vi "CreateEventTypeEnum.vi"() -> ()   [LabVIEW 2024]
uses:
  <vilib>/Utility/error.llb/Trim Whitespace One-Sided.vi
  SDL3/Events/EventType--enum.ctl
  <vilib>/regexp/Match Regular Expression.xnode
  SDL3/Events/Events.lvlib
panel:
  out "delimited string":string
  in  "#Define list":string="SDL_EVENT_QUIT           = 0x100, /**< User-requested quit */\n\n\n    SDL_EVENT_LOCALE_CHANGED,  /**< The user's locale preferences have changed. */\n\n    SDL_EVENT_SYSTEM_THEME_CHANGED, /**< The system theme changed */\n\n    SDL_EVENT_DISPLAY_ORIENTATION = 0x151,   /**< Display orientation has changed to data1 */\n    SDL_EVENT_DISPLAY_ADDED,                 /**< Display has been added to the system */\n    SDL_EVENT_DISPLAY_REMOVED,               /**< Display has been removed from the system */\n    SDL_EVENT_DISPLAY_MOVED,                 /**< Display has changed position */\n    SDL_EVENT_DISPLAY_DESKTOP_MODE_CHANGED,  /**< Display has changed desktop mode */\n    SDL_EVENT_DISPLAY_CURRENT_MODE_CHANGED,  /**< Display has changed current mode */\n    SDL_EVENT_DISPLAY_CONTENT_SCALE_CHANGED, /**< Display has changed content scale */\n\n\n\n    SDL_EVENT_WINDOW_SHOWN = 0x202,     /**< Window has been shown */\n    SDL_EVENT_WINDOW_HIDDEN,            /**< Window has been hidden */\n    SDL_EVENT_WINDOW_EXPOSED,           /**< Window has been exposed and should be redrawn, and can be redrawn directly from event watchers for this event */\n    SDL_EVENT_WINDOW_MOVED,             /**< Window has been moved to data1, data2 */\n    SDL_EVENT_WINDOW_RESIZED,           /**< Window has been resized to data1xdata2 */\n    SDL_EVENT_WINDOW_PIXEL_SIZE_CHANGED,/**< The pixel size of the window has changed to data1xdata2 */\n    SDL_EVENT_WINDOW_METAL_VIEW_RESIZED,/**< The pixel size of a Metal view associated with the window has changed */\n    SDL_EVENT_WINDOW_MINIMIZED,         /**< Window has been minimized */\n    SDL_EVENT_WINDOW_MAXIMIZED,         /**< Window has been maximized */\n    SDL_EVENT_WINDOW_RESTORED,          /**< Window has been restored to normal size and position */\n    SDL_EVENT_WINDOW_MOUSE_ENTER,       /**< Window has gained mouse focus */\n    SDL_EVENT_WINDOW_MOUSE_LEAVE,       /**< Window has lost mouse focus */\n    SDL_EVENT_WINDOW_FOCUS_GAINED,      /**< Window has gained keyboard focus */\n    SDL_EVENT_WINDOW_FOCUS_LOST,        /**< Window has lost keyboard focus */\n    SDL_EVENT_WINDOW_CLOSE_REQUESTED,   /**< The window manager requests that the window be closed */\n    SDL_EVENT_WINDOW_HIT_TEST,          /**< Window had a hit test that wasn't SDL_HITTEST_NORMAL */\n    SDL_EVENT_WINDOW_ICCPROF_CHANGED,   /**< The ICC profile of the window's display has changed */\n    SDL_EVENT_WINDOW_DISPLAY_CHANGED,   /**< Window has been moved to display data1 */\n    SDL_EVENT_WINDOW_DISPLAY_SCALE_CHANGED, /**< Window display scale has been changed */\n    SDL_EVENT_WINDOW_SAFE_AREA_CHANGED, /**< The window safe area has been changed */\n    SDL_EVENT_WINDOW_OCCLUDED,          /**< The window has been occluded */\n    SDL_EVENT_WINDOW_ENTER_FULLSCREEN,  /**< The window has entered fullscreen mode */\n    SDL_EVENT_WINDOW_LEAVE_FULLSCREEN,  /**< The window has left fullscreen mode */\n    SDL_EVENT_WINDOW_DESTROYED,         /**< The window with the associated ID is being or has been destroyed. If this message is being handled in an event watcher, the window handle is still valid and can still be used to retrieve any properties associated with the window. Otherwise, the handle has already been destroyed and all resources associated with it are invalid */\n    SDL_EVENT_WINDOW_HDR_STATE_CHANGED, /**< Window HDR properties have changed */\n\n\n\n    SDL_EVENT_KEY_DOWN        = 0x300, /**< Key pressed */\n    SDL_EVENT_KEY_UP,                  /**< Key released */\n    SDL_EVENT_TEXT_EDITING,            /**< Keyboard text editing (composition) */\n    SDL_EVENT_TEXT_INPUT,              /**< Keyboard text input */\n    SDL_EVENT_KEYMAP_CHANGED,          /**< Keymap changed due to a system event such as an input language or keyboard layout change. */\n    SDL_EVENT_KEYBOARD_ADDED,          /**< A new keyboard has been inserted into the system */\n    SDL_EVENT_KEYBOARD_REMOVED,        /**< A keyboard has been removed */\n    SDL_EVENT_TEXT_EDITING_CANDIDATES, /**< Keyboard text editing candidates */\n\n\n    SDL_EVENT_MOUSE_MOTION    = 0x400, /**< Mouse moved */\n    SDL_EVENT_MOUSE_BUTTON_DOWN,       /**< Mouse button pressed */\n    SDL_EVENT_MOUSE_BUTTON_UP,         /**< Mouse button released */\n    SDL_EVENT_MOUSE_WHEEL,             /**< Mouse wheel motion */\n    SDL_EVENT_MOUSE_ADDED,             /**< A new mouse has been inserted into the system */\n    SDL_EVENT_MOUSE_REMOVED,           /**< A mouse has been removed */\n\n\n    SDL_EVENT_JOYSTICK_AXIS_MOTION  = 0x600, /**< Joystick axis motion */\n    SDL_EVENT_JOYSTICK_BALL_MOTION,          /**< Joystick trackball motion */\n    SDL_EVENT_JOYSTICK_HAT_MOTION,           /**< Joystick hat position change */\n    SDL_EVENT_JOYSTICK_BUTTON_DOWN,          /**< Joystick button pressed */\n    SDL_EVENT_JOYSTICK_BUTTON_UP,            /**< Joystick button released */\n    SDL_EVENT_JOYSTICK_ADDED,                /**< A new joystick has been inserted into the system */\n    SDL_EVENT_JOYSTICK_REMOVED,              /**< An opened joystick has been removed */\n    SDL_EVENT_JOYSTICK_BATTERY_UPDATED,      /**< Joystick battery level change */\n    SDL_EVENT_JOYSTICK_UPDATE_COMPLETE,      /**< Joystick update is complete */\n\n\n    SDL_EVENT_GAMEPAD_AXIS_MOTION  = 0x650, /**< Gamepad axis motion */\n    SDL_EVENT_GAMEPAD_BUTTON_DOWN,          /**< Gamepad button pressed */\n    SDL_EVENT_GAMEPAD_BUTTON_UP,            /**< Gamepad button released */\n    SDL_EVENT_GAMEPAD_ADDED,                /**< A new gamepad has been inserted into the system */\n    SDL_EVENT_GAMEPAD_REMOVED,              /**< A gamepad has been removed */\n    SDL_EVENT_GAMEPAD_REMAPPED,             /**< The gamepad mapping was updated */\n    SDL_EVENT_GAMEPAD_TOUCHPAD_DOWN,        /**< Gamepad touchpad was touched */\n    SDL_EVENT_GAMEPAD_TOUCHPAD_MOTION,      /**< Gamepad touchpad finger was moved */\n    SDL_EVENT_GAMEPAD_TOUCHPAD_UP,          /**< Gamepad touchpad finger was lifted */\n    SDL_EVENT_GAMEPAD_SENSOR_UPDATE,        /**< Gamepad sensor was updated */\n    SDL_EVENT_GAMEPAD_UPDATE_COMPLETE,      /**< Gamepad update is complete */\n    SDL_EVENT_GAMEPAD_STEAM_HANDLE_UPDATED,  /**< Gamepad Steam handle has changed */\n\n\n    SDL_EVENT_FINGER_DOWN      = 0x700,\n    SDL_EVENT_FINGER_UP,\n    SDL_EVENT_FINGER_MOTION,\n\n\n\n\n    SDL_EVENT_CLIPBOARD_UPDATE = 0x900, /**< The clipboard or primary selection changed */\n\n\n    SDL_EVENT_DROP_FILE        = 0x1000, /**< The system requests a file open */\n    SDL_EVENT_DROP_TEXT,                 /**< text/plain drag-and-drop event */\n    SDL_EVENT_DROP_BEGIN,                /**< A new set of drops is beginning (NULL filename) */\n    SDL_EVENT_DROP_COMPLETE,             /**< Current set of drops is now complete (NULL filename) */\n    SDL_EVENT_DROP_POSITION,             /**< Position while moving over the window */\n\n\n    SDL_EVENT_AUDIO_DEVICE_ADDED = 0x1100,  /**< A new audio device is available */\n    SDL_EVENT_AUDIO_DEVICE_REMOVED,         /**< An audio device has been removed. */\n    SDL_EVENT_AUDIO_DEVICE_FORMAT_CHANGED,  /**< An audio device's format has been changed by the system. */\n\n\n    SDL_EVENT_SENSOR_UPDATE = 0x1200,     /**< A sensor was updated */\n\n\n    SDL_EVENT_PEN_PROXIMITY_IN = 0x1300,  /**< Pressure-sensitive pen has become available */\n    SDL_EVENT_PEN_PROXIMITY_OUT,          /**< Pressure-sensitive pen has become unavailable */\n    SDL_EVENT_PEN_DOWN,                   /**< Pressure-sensitive pen touched drawing surface */\n    SDL_EVENT_PEN_UP,                     /**< Pressure-sensitive pen stopped touching drawing surface */\n    SDL_EVENT_PEN_BUTTON_DOWN,            /**< Pressure-sensitive pen button pressed */\n    SDL_EVENT_PEN_BUTTON_UP,              /**< Pressure-sensitive pen button released */\n    SDL_EVENT_PEN_MOTION,                 /**< Pressure-sensitive pen is moving on the tablet */\n    SDL_EVENT_PEN_AXIS,                   /**< Pressure-sensitive pen angle/pressure/etc changed */\n\n\n    SDL_EVENT_CAMERA_DEVICE_ADDED = 0x1400,  /**< A new camera device is available */\n    SDL_EVENT_CAMERA_DEVICE_REMOVED,         /**< A camera device has been removed. */\n    SDL_EVENT_CAMERA_DEVICE_APPROVED,        /**< A camera device has been approved for use by the user. */\n    SDL_EVENT_CAMERA_DEVICE_DENIED,          /**< A camera device has been denied for use by the user. */\n\n\n    SDL_EVENT_RENDER_TARGETS_RESET = 0x2000, /**< The render targets have been reset and their contents need to be updated */\n    SDL_EVENT_RENDER_DEVICE_RESET, /**< The device has been reset and all textures need to be recreated */\n\n\n    SDL_EVENT_POLL_SENTINEL = 0x7F00, /**< Signals the end of an event poll cycle */\n\n   \n    SDL_EVENT_USER    = 0x8000  /** Events SDL_EVENT_USER through SDL_EVENT_LAST are for your use, and should be allocated with SDL_RegisterEvents()*/"
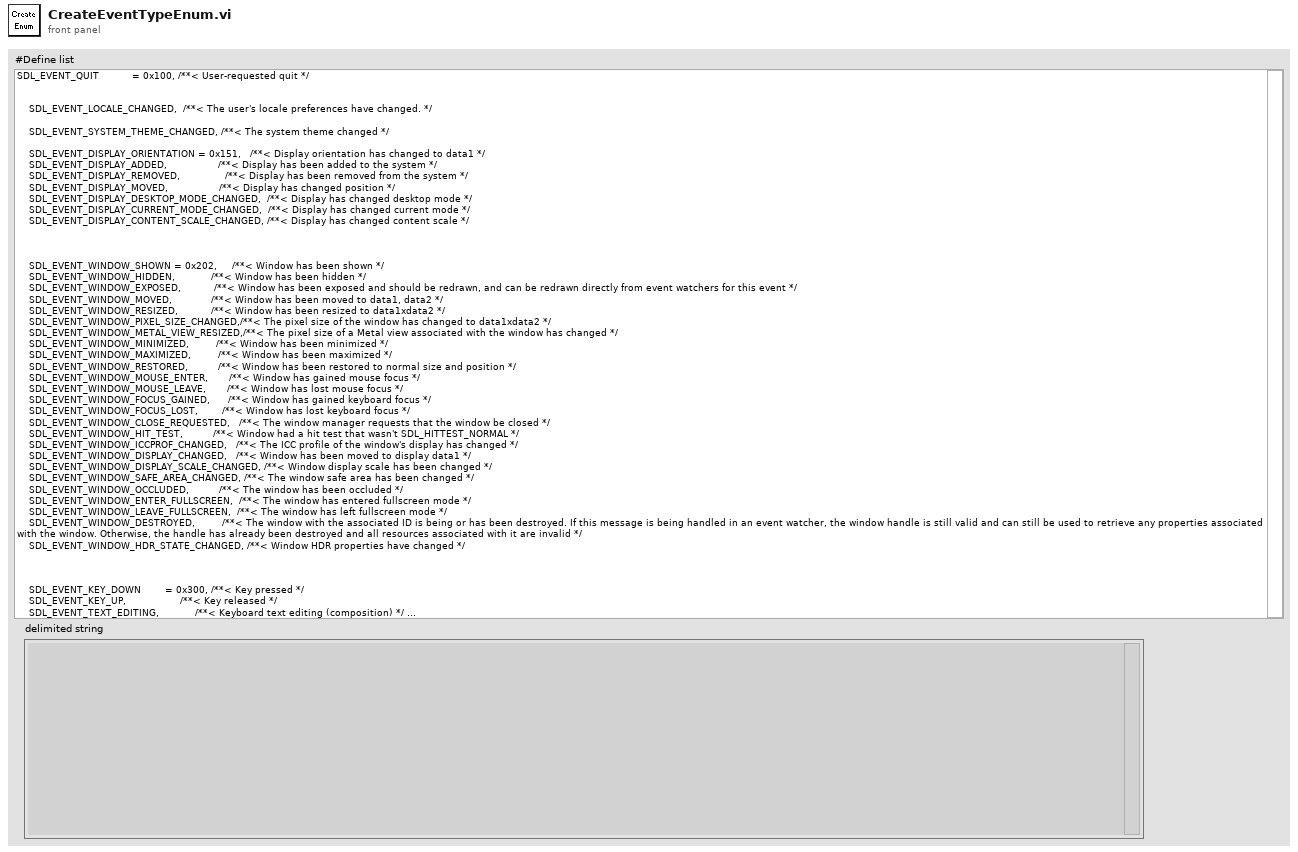
[diagram p1: front panel]
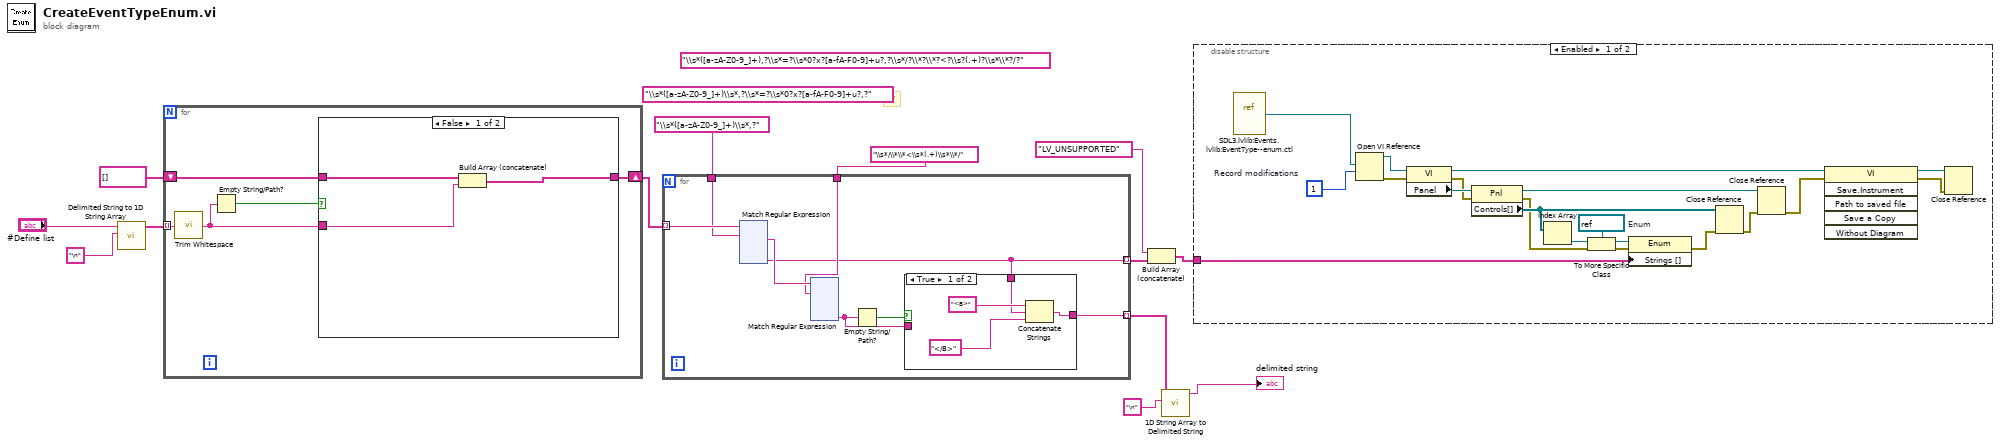
[diagram p0: block diagram]
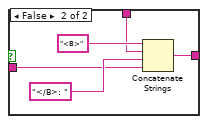
[diagram p4: hidden frame]
diagram:
  (unwired) "\\s*([a-zA-Z0-9_]+)\\s*,?\\s*=?\\s*0?x?[a-fA-F0-9]+u?,?" ("regular expression")
  (unwired) "\\s*([a-zA-Z0-9_]+),?\\s*=?\\s*0?x?[a-fA-F0-9]+u?,?\\s*/?\\*?\\*?<?\\s?(.+)?\\s*\\*?/?" ("regular expression")
  # "\\*/"
  n1 = call <vilib>:"Delimited String to 1D String Array.vi"("delimiter"="\n", "delimited string"="#Define list") -> ("string array"=w11:string[])  [unwired: 9 in]
  n2 = for {
    tunnel: w11 -> [w16] mode=indexing
    shift-right: [w17] -> w9
    shift-left: string[] [] -> [w18]
    n3 = call <vilib>:"Trim Whitespace.vi"("string"=w16) -> ("trimmed string"=w14:string)  [unwired: 1 in]
    n4 = Empty String/Path?(string/path=w14) -> (empty?=w15:bool)
    n5 = case shown="False" w15 {
      tunnel: w18 -> [w21 w22]
      tunnel: [w20 w22] -> w17
      tunnel: w14 -> [w19 _]
      frame False {
        n6 = Build Array (concatenate)(w21, w19) -> (w20:string[])
      }
      frame True {
      }
    }
  }
  n7 = for {
    tunnel: w9 -> [w30] mode=indexing
    tunnel: [w26] -> w8 mode=indexing
    tunnel: "\\s*([a-zA-Z0-9_]+)\\s*,?" ("regular expression") -> [w29]
    tunnel: [w23] -> w5 mode=indexing
    tunnel: "\\s*/\\*\\*<\\s*(.+)\\s*\\*/" ("regular expression") -> [w27]
    n8 = xnode "Match Regular Expression"("input string"=w30, "regular expression"=w29) -> ("after match"=w28:string, "submatch 1"=w26:string)  [unwired: 4 in, 4 out]
    n9 = xnode "Match Regular Expression"("input string"=w28, "regular expression"=w27) -> ("submatch 1"=w25:string)  [unwired: 4 in, 5 out]
    n10 = Empty String/Path?(string/path=w25) -> (empty?=w24:bool)
    n11 = case shown="True" w24 {
      tunnel: w26 -> [w32 w37]
      tunnel: w25 -> [_ w36]
      tunnel: [w31 w35] -> w23
      frame True {
        n12 = Concatenate Strings("<B>" ("string"), w32, "</B>" ("string")) -> (w31:string)
      }
      frame False {
        n13 = Concatenate Strings("<B>" ("string"), w37, "</B>: " ("string"), w36) -> (w35:string)
      }
    }
  }
  n14 = Build Array (concatenate)("LV_UNSUPPORTED" ("regular expression"), w8) -> (w2:string[])
  n15 = call <vilib>:"1D String Array to Delimited String.vi"("delimiter"="\n", "string array"=w5) -> ("delimited string"=→"delimited string":string)  [unwired: 9 in]
  n16 = disable-structure shown="Enabled" {
    disable-tunnel: w2 -> [w279 _]
    frame Enabled {
      w289 = refnum<vi> refnum  # Enum
      w295 = 1  # Record modifications
      n17 = vi-ref "SDL3.lvlib:Events.lvlib:EventType--enum.ctl"() -> (w296:refnum<vi>)
      n18 = Open VI Reference(vi path=w296, options=w295) -> (vi reference=w294:refnum<vi>, error out=w297:errorcluster)  [unwired: 4 in]
      n19 = property class="VI"(reference=w294, error in=w297) -> (reference out=w284:refnum<vi>, error out=w292:errorcluster, "Panel"=w293:refnum<vi>)
      n20 = property class="Pnl"(reference=w293, error in=w292) -> (reference out=w291:refnum<vi>, error out=w282:errorcluster, "Controls[]"=w287:refnum<vi>[])
      n21 = Index Array(array=w287) -> (element=w288:refnum<vi>)  [unwired: 1 in]
      n22 = To More Specific Class(target class=w289, reference=w288, error in=w282) -> (specific class reference=w281:refnum<vi>, error out=w280:errorcluster)
      n23 = property class="Enum"(reference=w281, error in=w280, "Strings []"=w279) -> (error out=w278:errorcluster)  [unwired: 1 out]
      n24 = Close Reference(reference=w287, error in (no error)=w278) -> (error out=w286:errorcluster)
      n25 = Close Reference(reference=w291, error in (no error)=w286) -> (error out=w290:errorcluster)
      n26 = invoke class="VI" method="Save.Instrument"(reference=w284, error in=w290) -> (reference out=w283:refnum<vi>, error out=w285:errorcluster)  [unwired: 4 in, 4 out]
      n27 = Close Reference(reference=w283, error in (no error)=w285) -> ()  [unwired: 1 out]
    }
    frame Disabled {
    }
  }
